vi "checkBeginPreparePenaltyAllyPlay.vi"(8 "error in (no error)":errorcluster, 9 "last command_interpreted":T1, 10 "Game":refnum<class "Game.lvclass">, 11 "PreparePenaltyAllyPlay in":refnum<class "PreparePenaltyAllyPlay.lvclass">) -> (0 "error out":errorcluster, 2 "Boolean":bool, 3 "PreparePenaltyAllyPlay out":refnum<class "PreparePenaltyAllyPlay.lvclass">)   [LabVIEW 2023, in "PreparePenaltyAllyPlay.lvclass"]
uses:
  PreparePenaltyAllyPlay.lvclass
  Game_class/Game.lvclass
  Referee_class/command_interpreted.ctl
  Game_class/Game.lvclass/Game.ctl
  Referee_class/Referee.lvclass/Referee.ctl
  Game_class/Read Referee.vi
  Game_class/Read EventsRef.vi
  Referee_class/Read command_interpreted.vi
  Referee_class/Referee.lvclass
  Events_class/Events.lvclass
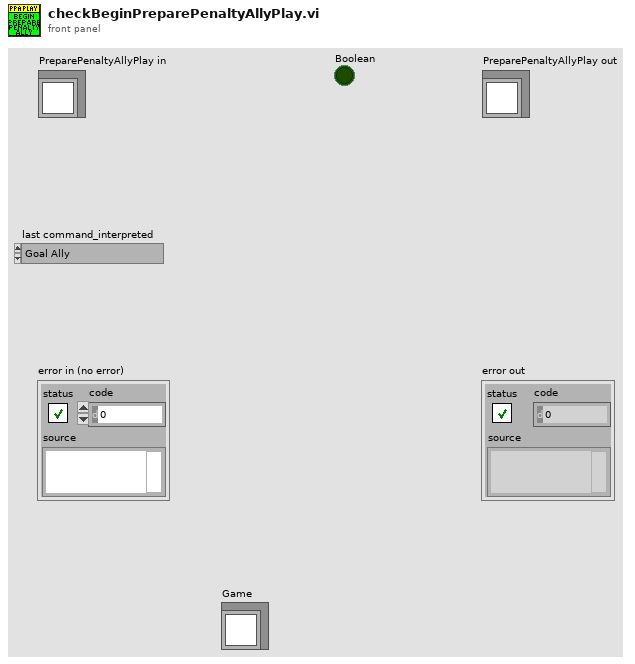
[diagram p1: front panel]
types:
  T1 = typedef "command_interpreted.ctl" = enum16{"Goal Ally", "Goal Enemy", "Ball Placement Enemy", "Ball Placement Ally", "Normal Half Time", "Extra Time  Break", "Extra Half Time", "None", "Post Game", "PKA Normal Start", "Prepare Kickoff Ally", "PKE Normal Start", "Prepare Kickoff Enemy", "Force Start", "Halt", "Timeout", "Prepare Penalty Ally", "Prepare Penalty Enemy", "PPA NormalStart", "PPE Normal Start", "Indirect Free Ally", "Direct Free Enemy", "Direct Free Ally", "Indirect Free Enemy", "Stop"}
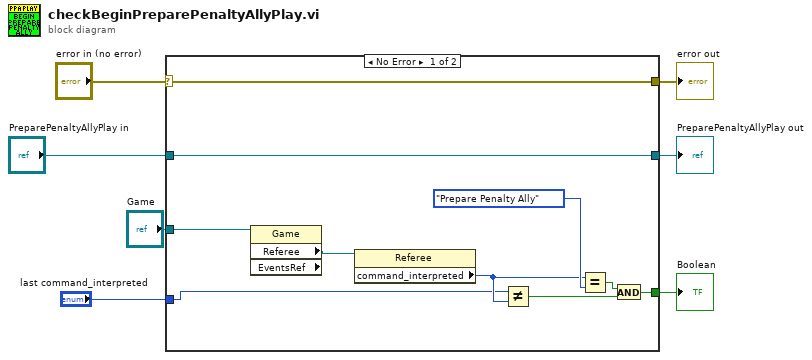
[diagram p0: block diagram]
diagram:
  n1 = case shown="No Error" "error in (no error)" {
    selector: "error in (no error)" -> [w16 w19]
    tunnel: [w16 w19] -> w6
    tunnel: [w17 w18] -> w4
    tunnel: "PreparePenaltyAllyPlay in" -> [w17 w18]
    tunnel: "Game" -> [w10 _]
    tunnel: [w9 _] -> w2
    tunnel: "last command_interpreted" -> [w8 _]
    frame No Error {
      n2 = property class="Game" props=["Referee", "EventsRef"](reference=w10) -> ("Referee"=w15:refnum<class "Referee.lvclass">)  [unwired: 1 in, 3 out]
      n3 = property class="Referee"(reference=w15) -> ("command_interpreted"=w12:T1)  [unwired: 1 in, 2 out]
      n4 = Not Equal?(x=w8, y=w12) -> (x != y?=w11:bool)
      n5 = Equal?(x=w12, y=command_interpreted."Prepare Penalty Ally" ("command_interpreted")) -> (x = y?=w13:bool)
      n6 = And(x=w13, y=w11) -> (x .and. y?=w9:bool)
    }
    frame Error {
    }
  }
  "error out" <- w6
  "PreparePenaltyAllyPlay out" <- w4
  "Boolean" <- w2
